vi "Set Connected.vi"(10 "Connected":bool, 11 "TCP Process in":refnum<class "TCP Process.lvclass">) -> (3 "TCP Process out":refnum<class "TCP Process.lvclass">)   [LabVIEW 2019, in "TimingDRV Engine.lvlib" / "TCP Process.lvclass"]
uses:
  TCP Process.lvclass
  TCP Process.lvclass/TCP Process.ctl
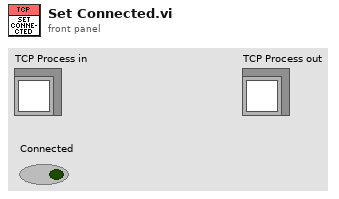
[diagram p1: front panel]
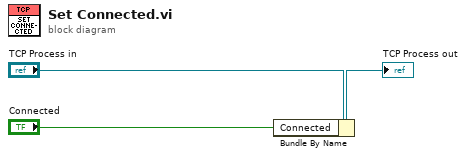
[diagram p0: block diagram]
diagram:
  n1 = Bundle By Name(cluster="TCP Process in", "Connected"="Connected") -> (→"TCP Process out":refnum<class "TCP Process.lvclass">)
